vi "Stepper Wait for Move.vi"(0 "Instrument Address":refnum<visa-resource-name>, 1 "Motor Number":u32=1 min=1 max=255 step=1, 3 "error in (no error)":errorcluster) -> (5 "error out":errorcluster)   [LabVIEW 2024]
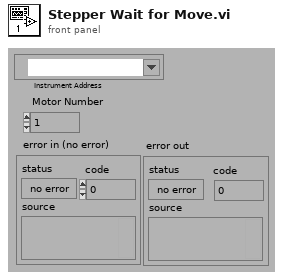
[diagram p1: front panel]
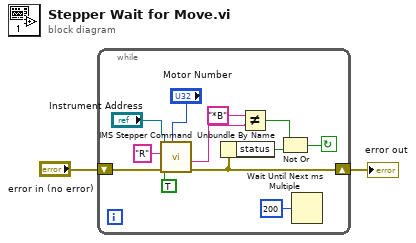
[diagram p0: block diagram]
diagram:
  n1 = while {
    shift-left: "error in (no error)" -> [w10]
    shift-right: [w9] -> w1
    stop <- w8 continue-if-true
    n2 = call "IMS Stepper Command.vi"("Motor Number"="Motor Number", "error in (no error)"=w10, "Mode"=TRUE, "Command"="R", "Instrument Address"="Instrument Address") -> ("error out"=w9:errorcluster, "Response"=w6:string)  [unwired: 1 in, 2 out]
    n3 = Unbundle By Name(w9) -> ("status"=w7:bool)
    n4 = Not Equal?(x="*B", y=w6) -> (x != y?=w4:bool)
    n5 = Not Or(1:w7, 2:w4) -> (0:w8:bool)
    n6 = Wait Until Next ms Multiple(millisecond multiple=u32 200) -> ()  [unwired: 1 out]
  }
  "error out" <- w1
